vi "Log State Change.vi"(8 "error in (no error)":errorcluster, 10 "Command":T1, 11 "CIFCorePlugin in":refnum<class "CIFCorePlugin.lvclass">) -> (0 "error out":errorcluster, 3 "CIFCorePlugin out":refnum<class "CIFCorePlugin.lvclass">)   [LabVIEW 2021, in "CIFCorePlugin.lvclass"]
uses:
  CIFCorePlugin.lvclass
  CIFCorePlugin.lvclass/CIFCorePlugin.ctl
  Accessors/Read Plugin Name.vi
  Accessors/Read gRPC Server Port.vi
  Accessors/Read Version.vi
  CIFUtilities/CIFLogs/CIFLogs.lvlib
  CIFUtilities/CIFLogs/Typedef/Plugin State Commands.ctl
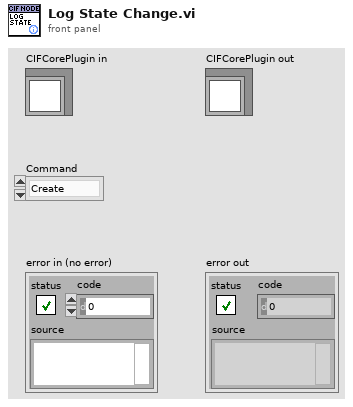
[diagram p1: front panel]
types:
  T1 = typedef "Plugin State Commands.ctl" = enum16{"Create", "Run", "Pause", "Destroy"}
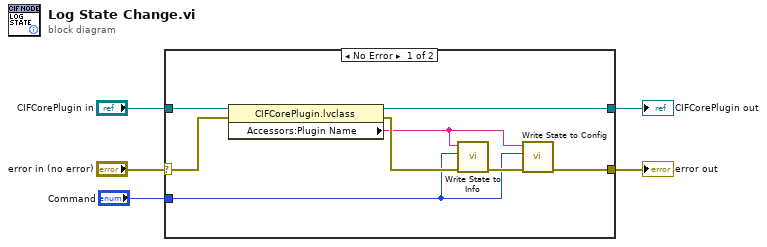
[diagram p0: block diagram]
diagram:
  n1 = case shown="No Error" "error in (no error)" {
    selector: "error in (no error)" -> [w10 w15]
    tunnel: [w6 w15] -> w4
    tunnel: [w12 w14] -> w2
    tunnel: "CIFCorePlugin in" -> [w13 w14]
    tunnel: "Command" -> [w8 _]
    frame No Error {
      n2 = property class="CIFCorePlugin.lvclass"(reference=w13, error in=w10) -> (reference out=w12:refnum<class "CIFCorePlugin.lvclass">, error out=w11:errorcluster, "Accessors:Plugin Name"=w7:string)
      n3 = call "Write State to Info.vi"("error in (no error)"=w11, "Command"=w8, "Plugin Name"=w7) -> ("error out"=w9:errorcluster)  [unwired: 8 in]
      n4 = call "Write State to Config.vi"("error in (no error)"=w9, "Command"=w8, "Plugin Name"=w7) -> ("error out"=w6:errorcluster)  [unwired: 8 in]
    }
    frame Error {
    }
  }
  "error out" <- w4
  "CIFCorePlugin out" <- w2
